vi "PH_ImageCoG_Plotter.PC Read Cali Data.vi"(0 "i ref in":refnum<vi>, 5 "error in (no error)":errorcluster) -> (14 "i ref out":refnum<vi>, 19 "error out":errorcluster)   [LabVIEW 2014, in "PH_ImageCoG_Plotter.lvlib"]
doc: "This VI reads the calibration data file and sets the own attributes."
uses:
  PH_ImageCoG_Plotter.lvlib
  PH_ImageCalibrator/PH_ImageCalibrator.Calibration Data.ctl
  PH_StatusHandler/PH_StatusHandler.Status.ctl
  PH_Common/PH_Common.lvlib
  PH_ImageCalibrator/PH_ImageCalibrator.lvlib
  PH_StatusHandler/PH_StatusHandler.lvlib
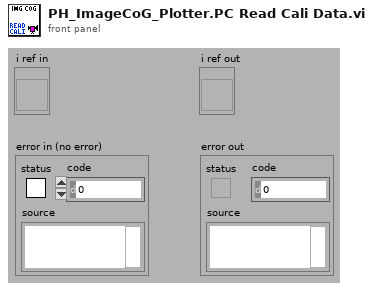
[diagram p1: front panel]
types:
  T1 = typedef "PH_ImageCalibrator.lvlib/PH_ImageCalibrator.Calibration Data.ctl" = cluster{"Date":string, "Time":string, "Cam Settings":cluster{"Cam ID":string, "Gain":dbl, "Brightness":dbl, "Shutter":dbl, "Cam Error":bool, "Mode":i32}, "Background Image":cluster{"Image":dbl[][], "Image Error":bool}, "Linear Calibration":cluster{"Calibration Factor":dbl, "not mm or mrad":bool}, "Energy Calibration":cluster{"Calibration Factor":dbl, "no mJ":bool}}
  T2 = typedef "PH_ImageCoG_Plotter.lvlib/PH_ImageCoG_Plotter.i attribute.ctl" = cluster{"GUI Refs":cluster{"Delete":refnum<vi>, "Calibration status":refnum<vi>, "BI subtracted":refnum<vi>, "calc Beam Anal":refnum<vi>, "CoG - x":refnum<vi>, "CoG - y":refnum<vi>, "Type":refnum<vi>, "Center":refnum<vi>, "exp - X":refnum<vi>, "exp - Y":refnum<vi>, "Delta - X":refnum<vi>, "Delta - Y":refnum<vi>, "Available Cams":refnum<vi>, "CoG X":refnum<vi>, "CoG Y":refnum<vi>, "Delta X":refnum<vi>, "Delta Y":refnum<vi>, "Export Data":refnum<vi>, "Calibration data":refnum<vi>}, "Calibration":cluster{"Status":T3, "Calibration data":T1, "Calibration Data File":path}, "Beam Analysis":cluster{"on":bool, "exp - X":i32, "exp - Y":i32, "Type":bool, "Data":cluster{"current time":timestamp, "CoG-x":dbl, "CoG-y":dbl, "Delta-x":dbl, "Delta-y":dbl}[], "Datasets strored":i32, "Dataarray Size":i32}, "Cam instances":string[], "DIM Service Events":T4[], "Images":cluster{"Background":T7, "OP":T7, "GUI":T7}}
  T3 = typedef "PH_StatusHandler.lvlib/PH_StatusHandler.Status.ctl" = i16
  T4 = typedef "BaseProcess.lvlib/BaseProcess.event definition.ctl" = cluster{"CAEEvtDef":T5, "Data Descriptor":T6}
  T5 = typedef "CAEObj.lvlib/CAEObj.event definition.ctl" = cluster{"URL":string, "enable":bool, "ignoreResID":bool}
  T6 = typedef "BaseProcess.lvlib/BaseProcess.descriptor string definition.ctl" = string
  T7 = typedef "IMAQ Image.ctl" = refnum<image>
  T8 = cluster{"Cam ID":string, "Gain":dbl, "Brightness":dbl, "Shutter":dbl, "Cam Error":bool, "Mode":i32}
  T9 = cluster{"Calibration Factor":dbl, "not mm or mrad":bool}
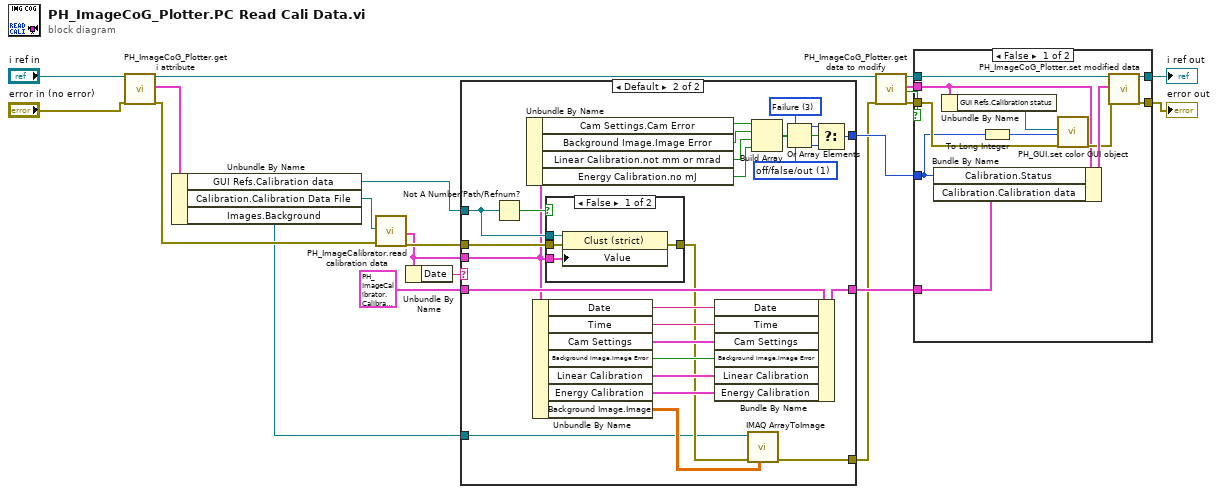
[diagram p0: block diagram]
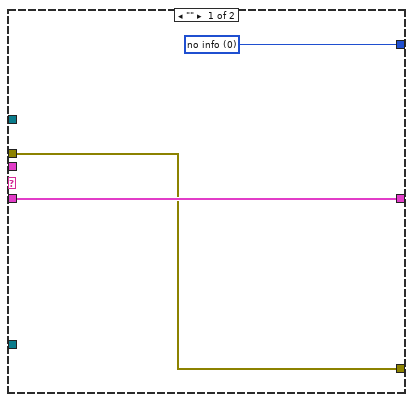
[diagram p3: hidden frame]
diagram:
  n1 = call "PH_ImageCoG_Plotter.get i attribute.vi"("i ref in"="i ref in", "error in (no error)"="error in (no error)") -> ("i ref out"=w15:refnum<vi>, "i attribute"=w18:T2, "error out"=w19:errorcluster)  [unwired: 15 in]
  n2 = Unbundle By Name(w18) -> ("GUI Refs.Calibration data"=w21:refnum<vi>, "Calibration.Calibration Data File"=w1:path, "Images.Background"=w5:T7)
  n3 = call "PH_ImageCalibrator.read calibration data.vi"("Calibration Data File"=w1, "error in (no error)"=w19) -> ("Calibration data"=w3:T1, "error out"=w20:errorcluster)  [unwired: 16 in]
  n4 = Unbundle By Name(w3) -> ("Date"=w2:string)
  n5 = case shown="Default" w2 {
    tunnel: w3 -> [_ w26]
    tunnel: w20 -> [w22 w49]
    tunnel: w21 -> [_ w48]
    tunnel: [w24 w39] -> w8
    tunnel: [w23 w36] -> w7
    tunnel: T1 {"Date"="", "Time"="", "Cam Settings"={"Cam ID"="N/A", "Gain"=0.0, "Brightness"=0.0, "Shutter"=0.0, "Cam Error"=FALSE, "Mode"=0}, "Background Image"={"Image"=[], "Image Error"=FALSE}, "Linear Calibration"={"Calibration Factor"=0.0, "not mm or mrad"=FALSE}, "Energy Calibration"={"Calibration Factor"=0.0, "no mJ"=FALSE}} ("Calibration data") -> [w23 w37]
    tunnel: w5 -> [_ w25]
    tunnel: [w22 w28] -> w4
    frame "" {
      w24 = T3 0 items=["no info", "off/false/out", "on/true/in", "Failure", "Alarm", "Status 1", "Status 2", "Status 3"]
    }
    frame Default {
      w38 = T3 3 items=["no info", "off/false/out", "on/true/in", "Failure", "Alarm", "Status 1", "Status 2", "Status 3"] ("t")
      w40 = T3 1 items=["no info", "off/false/out", "on/true/in", "Failure", "Alarm", "Status 1", "Status 2", "Status 3"]
      n6 = Not A Number/Path/Refnum?(number/path/refnum=w48) -> (NaN/Path/Refnum?=w47:bool)
      n7 = Unbundle By Name(w26) -> ("Cam Settings.Cam Error"=w46:bool, "Background Image.Image Error"=w45:bool, "Linear Calibration.not mm or mrad"=w44:bool, "Energy Calibration.no mJ"=w43:bool)
      n8 = Unbundle By Name(w26) -> ("Date"=w35:string, "Time"=w34:string, "Cam Settings"=w33:T8, "Background Image.Image Error"=w32:bool, "Linear Calibration"=w31:T9, "Energy Calibration"=w30:cluster{"Calibration Factor":dbl, "no mJ":bool}, "Background Image.Image"=w27:dbl[][])
      n9 = case shown="False" w47 {
        tunnel: w49 -> [w53 w54]
        tunnel: [w52 w54] -> w29
        tunnel: w48 -> [w51 _]
        tunnel: w26 -> [w50 _]
        frame False {
          n10 = property class="Clust (strict)"(reference=w51, error in=w53, "Value"=w50) -> (error out=w52:errorcluster)  [unwired: 1 out]
        }
        frame True {
        }
      }
      n11 = Bundle By Name(cluster=w37, "Date"=w35, "Time"=w34, "Cam Settings"=w33, "Background Image.Image Error"=w32, "Linear Calibration"=w31, "Energy Calibration"=w30) -> (w36:T1)
      n12 = call "IMAQ ArrayToImage"("Image Pixels (Float)"=w27, "error in (no error)"=w29, "Image"=w25) -> ("error out"=w28:errorcluster)  [unwired: 7 in, 1 out]
      n13 = Build Array(w46, w45, w44, w43) -> (w42:bool[])
      n14 = Or Array Elements(Boolean array=w42) -> (logical OR=w41:bool)
      n15 = Select(t=w38, s=w41, f=w40) -> (s? t:f=w39:T3)
    }
  }
  n16 = call "PH_ImageCoG_Plotter.get data to modify.vi"("i ref in"=w15, "error in (no error)"=w4) -> ("i ref out"=w13:refnum<vi>, "i attribute"=w9:T2, "timed out"=w11:bool, "error out"=w14:errorcluster)  [unwired: 14 in]
  n17 = case shown="False" w11 {
    tunnel: w14 -> [w60 w66]
    tunnel: w13 -> [w65 w67]
    tunnel: [w64 w67] -> w12
    tunnel: [w63 w66] -> w10
    tunnel: w9 -> [w58 _]
    tunnel: w8 -> [w56 _]
    tunnel: w7 -> [w61 _]
    frame False {
      n18 = Bundle By Name(cluster=w58, "Calibration.Status"=w56, "Calibration.Calibration data"=w61) -> (w62:T2)
      n19 = Unbundle By Name(w58) -> ("GUI Refs.Calibration status"=w57:refnum<vi>)
      n20 = To Long Integer(number=w56) -> (32bit integer=w55:i32)
      n21 = call "PH_GUI.set color GUI object.vi"("GUI object Ref"=w57, "State"=w55, "error in (no error)"=w60) -> ("error out"=w59:errorcluster)  [unwired: 16 in]
      n22 = call "PH_ImageCoG_Plotter.set modified data.vi"("i ref in"=w65, "i attribute"=w62, "error in (no error)"=w59) -> ("i ref out"=w64:refnum<vi>, "error out"=w63:errorcluster)  [unwired: 15 in]
    }
    frame True {
    }
  }
  "i ref out" <- w12
  "error out" <- w10
